vi "setAttributes.vi"(0 "reference":refnum<class "ClassNode.lvclass">, 1 "name":refnum<class "MultiLineString.lvclass">, 5 "error in (no error)":errorcluster) -> (14 "reference out":refnum<class "ClassNode.lvclass">, 19 "error out":errorcluster)   [LabVIEW 2016, in "ClassNode.lvclass"]
doc: "public void setAttributes(MultiLineString newValue)"
uses:
  <resource>/Framework/Providers/Open_GDS/UML/ClassNode_class/ClassNode.lvclass
  <resource>/Framework/Providers/Open_GDS/UML/MultiLineString_class/MultiLineString.lvclass
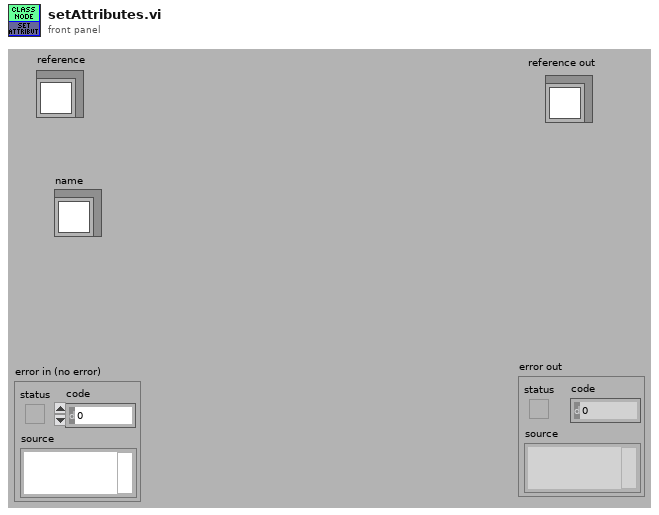
[diagram p1: front panel]
types:
  T1 = typedef "ClassNode.lvclass/ObjectAttributes.ctl" = cluster{"midHeight":dbl, "botHeight":dbl, "name":refnum<class "MultiLineString.lvclass">, "attributes":refnum<class "MultiLineString.lvclass">, "methods":refnum<class "MultiLineString.lvclass">, "DEFAULT_COMPARTMENT_HEIGHT":i32, "DEFAULT_WIDTH":i32, "DEFAULT_HEIGHT":i32, "showMethods":bool, "showAttributes":bool, "ClassPath":path}
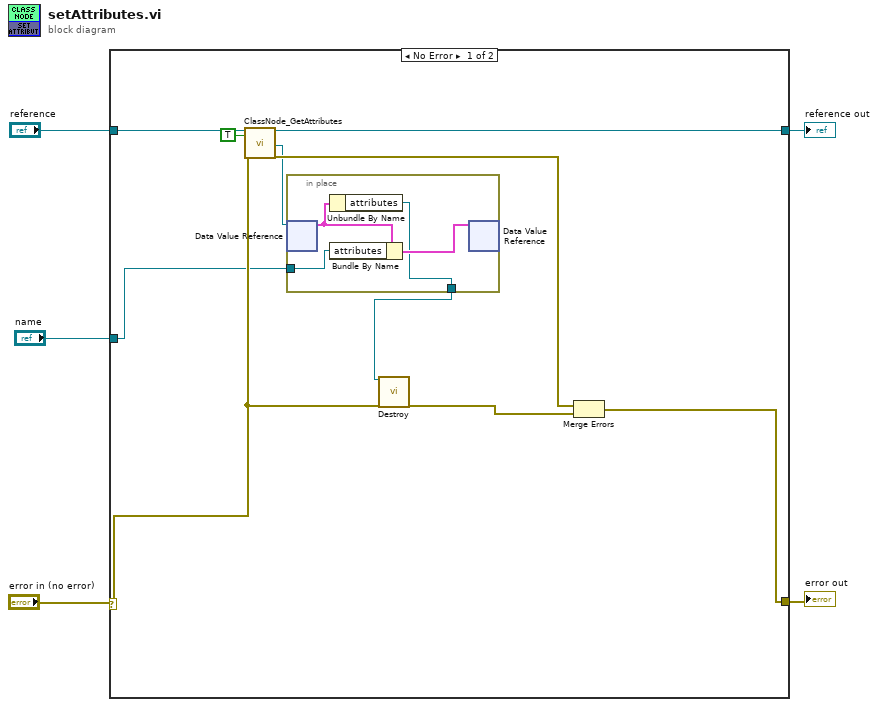
[diagram p0: block diagram]
diagram:
  n1 = case shown="No Error" "error in (no error)" {
    selector: "error in (no error)" -> [w12 w20]
    tunnel: "reference" -> [w15 w21]
    tunnel: [w14 w20] -> w4
    tunnel: [w13 w21] -> w3
    tunnel: "name" -> [w7 _]
    frame No Error {
      n2 = call <resource>:"ClassNode_GetAttributes.vi"("reference in"=w15, "OnlyGetDvrReference(False)"=TRUE, "error in (no error)"=w12) -> ("reference out"=w13:refnum<class "ClassNode.lvclass">, "DataRef"=w8:refnum<data-value>, "error out"=w10:errorcluster)  [unwired: 13 in, 1 out]
      n3 = in-place {
        in-place-border: w7 -> [w18]
        in-place-border: [w16] -> w6
        n4 = in-place-dvr #1(w8) -> (w19:T1)  [unwired: 1 out]
        n5 = Unbundle By Name(w19) -> ("attributes"=w16:refnum<class "MultiLineString.lvclass">)
        n6 = Bundle By Name(cluster=w19, "attributes"=w18) -> (w17:T1)
        n7 = in-place-dvr #1(w17) -> ()  [unwired: 2 out]
      }
      n8 = call-dynamic "Destroy.vi"("reference"=w6, "error in (no error)"=w12) -> ("error out"=w11:errorcluster)  [unwired: 17 out]
      n9 = Merge Errors(w10, w11) -> (w14:errorcluster)
    }
    frame Error {
    }
  }
  "reference out" <- w3
  "error out" <- w4
